vi "CheckForBinary.vi"(3 "Image in":T1 {"Dialogs" format="%.0b"}) -> (0 "Success?":bool)   [LabVIEW 2024]
doc: "This VI returns a boolean value depending upon whether the image input is binary or not. It also throws an error message to user."
uses:
  <userlib>/ImageProcessing/QTLIB_2595_LV86/QT_Image.ctl
  <userlib>/ImageProcessing/CameraGlobals.vi
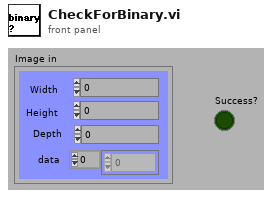
[diagram p1: front panel]
types:
  T1 = typedef "QT_Image.ctl" = cluster{"Width":i32, "Height":i32, "Depth":i32, "data":u8[], "Compressed data":u8[], "Color table":u32[], "Duration":i32, "Options":i32, "Timestamp":i32, "ID":i32, "Reserved":i32, "Dialogs":u32}
  T2 = typedef "QT_Ref.ctl" = refnum<k1>
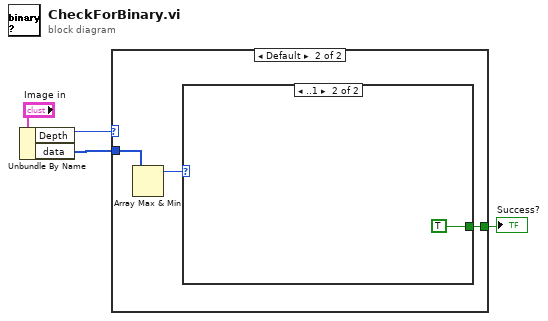
[diagram p0: block diagram]
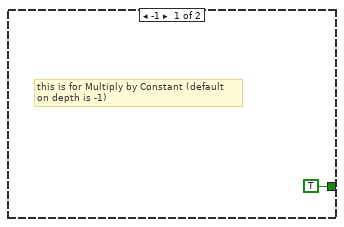
[diagram p2: hidden frame]
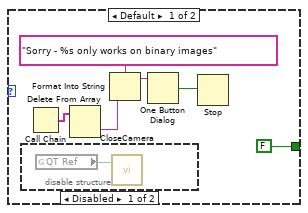
[diagram p3: hidden frame]
diagram:
  n1 = Unbundle By Name("Image in") -> ("Depth"=w1:i32, "data"=w2:u8[])
  n2 = case shown="Default" w1 {
    tunnel: [TRUE w8] -> w3
    tunnel: w2 -> [_ w7]
    frame -1 {
      # "this is for Multiply by Constant (default\non depth is -1)"
    }
    frame Default {
      n3 = Array Max & Min(array=w7) -> (max value=w6:u8)  [unwired: 3 out]
      n4 = case shown="..1" w6 {
        tunnel: [FALSE TRUE] -> w8
        frame Default {
          n5 = disable-structure shown="Disabled" {
            frame Disabled {
              n6 = global read "CameraGlobals.vi" "QT Ref"() -> (w15:T2)
              n7 = call <userlib>:"CloseCamera.vi"("QT Ref In"=w15) -> ()  [unwired: 2 in, 1 out]
            }
            frame Enabled {
            }
          }
          n8 = Call Chain() -> (call chain=w12:string[])
          n9 = Delete From Array(array=w12) -> (deleted portion=w11:string)  [unwired: 2 in, 1 out]
          n10 = Format Into String(format string="Sorry - %s only works on binary images" ("message"), w11) -> (resulting string=w13:string)  [unwired: 2 in, 1 out]
          n11 = One Button Dialog(message=w13) -> (true=w9:bool)  [unwired: 1 out]
          n12 = Stop(stop? (T)=w9) -> ()
        }
        frame ..1 {
        }
      }
    }
  }
  "Success?" <- w3
